vi "CreateSaturated.vi"() -> (2 "Golden":refnum<queue>, 3 "POTTypedCircularBuffer out":refnum<class "POTTypedCircularBuffer.lvclass">)   [LabVIEW 2024, in "POTCircularBuffer.Tests.Units.lvlib"]
uses:
  POTCircularBuffer.Tests.Units.lvlib
  POTTypedCircularBuffer.lvclass
  Type.ctl
  POTTypedCircularBuffer.lvclass/POTTypedCircularBuffer.ctl
  Wrap.vi
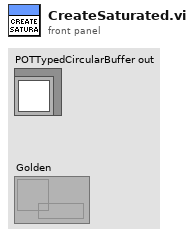
[diagram p1: front panel]
types:
  T1 = typedef "POTTypedCircularBuffer.lvclass/Type.ctl" = i32
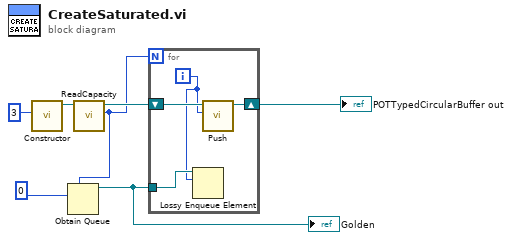
[diagram p0: block diagram]
diagram:
  n1 = call "Constructor.vi"("Capacity 2^n"=u32 3 ("Capacity")) -> ("POTTypedCircularBuffer out"=w6:refnum<class "POTTypedCircularBuffer.lvclass">)  [unwired: 10 in]
  n2 = call "ReadCapacity.vi"("POTTypedCircularBuffer in"=w6) -> ("capacity"=w2:i32, "POTTypedCircularBuffer out"=w5:refnum<class "POTTypedCircularBuffer.lvclass">)  [unwired: 9 in]
  n3 = Obtain Queue(max queue size (-1, unlimited)=w2, element data type=T1 0 ("Type")) -> (queue out=w1:refnum<queue>)  [unwired: 3 in, 2 out]
  "Golden" <- w1
  n4 = for {
    N: w2 -> [_]
    shift-right: [w10] -> w4
    shift-left: w5 -> [w11]
    tunnel: w1 -> [w9]
    i -> [w8]
    n5 = Lossy Enqueue Element(queue=w9, element=w8) -> ()  [unwired: 1 in, 4 out]
    n6 = call "Push.vi"("Element"=w8, "POTTypedCircularBuffer in"=w11) -> ("POTTypedCircularBuffer out"=w10:refnum<class "POTTypedCircularBuffer.lvclass">)  [unwired: 9 in]
  }
  "POTTypedCircularBuffer out" <- w4
